vi "Example_Manifold Learning.vi"() -> ()   [LabVIEW 2020]
uses:
  <vilib>/Utility/miscctls.llb/LV3DPointTypeDef.ctl
  <vilib>/addons/Machine Learning/Utilities/ml_Neighborhood Graph_Para.ctl
  <vilib>/addons/Machine Learning/Visualization/Visualization (3D).vi
  <vilib>/addons/Machine Learning/Visualization/Visualization (2D).vi
  <vilib>/addons/Machine Learning/NILabs_MLT.lvlib
panel:
  in  "# of samples":i32=1024
  in  "Data set":enum16{"swiss roll", "hemisphere", "3 balls"}(ring)=3
  in  "Algorithm":T1(ring)
  out "2-D Projections of the data":cluster{"X":dbl[], "Y":dbl[]}[](graph)
  out "error out":errorcluster
  out "3-D Data":refnum<vi>(3d-picture)
  # "Introduction:\nA list of dimension reduction algorithms can be selected to project several 3-D data to 2-D space. Some of the data sets (e.g., swiss roll) represent 2-D manifolds embedded in 3-D space. Their underlying structure can be correctly revealed in the projection when a suitable algorithm is selected."
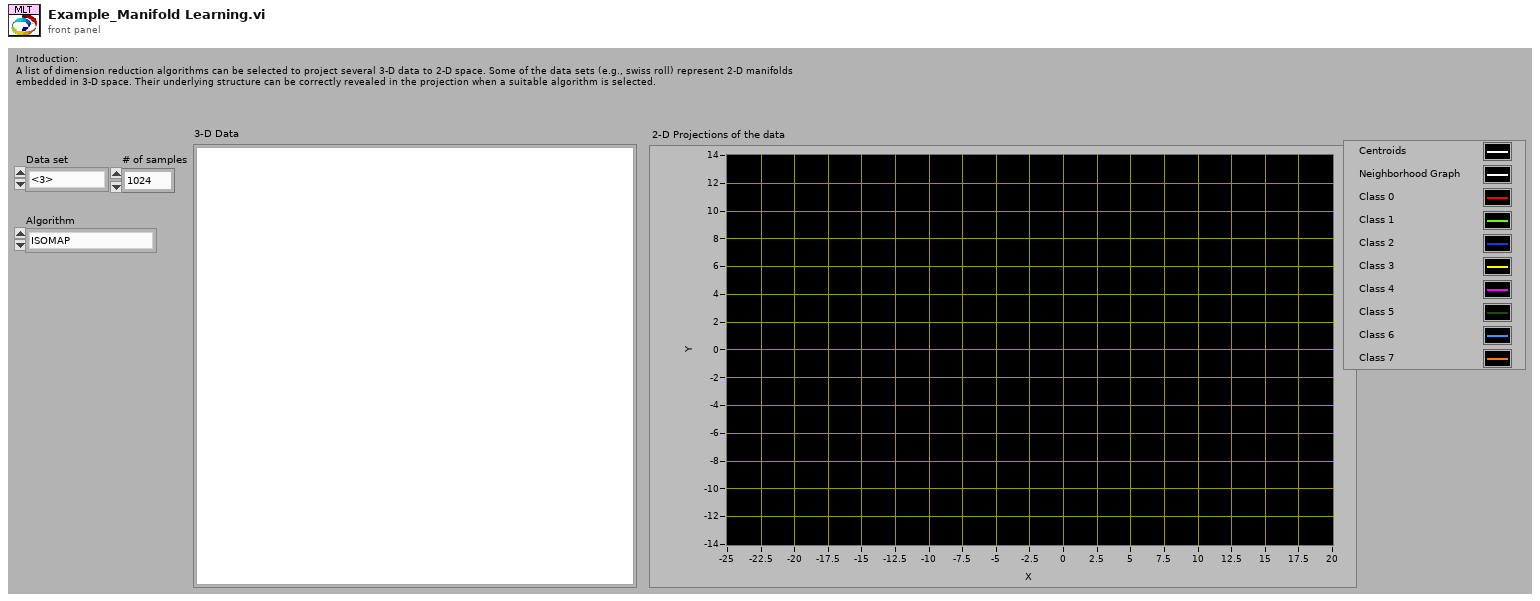
[diagram p1: front panel]
types:
  T1 = enum16{"ISOMAP", "Locally-Linear Embedding (LLE)", "PCA", "MDS", "LDA"}
  T2 = typedef "LV3DPointTypeDef.ctl" = cluster{"X":sgl, "Y":sgl, "Z":sgl}
  T3 = typedef "NILabs_MLT.lvlib/ml_Neighborhood Graph_Para.ctl" = cluster{"algorithm":enum16{"eps-Neighborhood Graph", "k-Nearest Neighbor Graph", "Mutual k-Nearest Neighbor Graph"}, "k":i32, "eps":dbl}
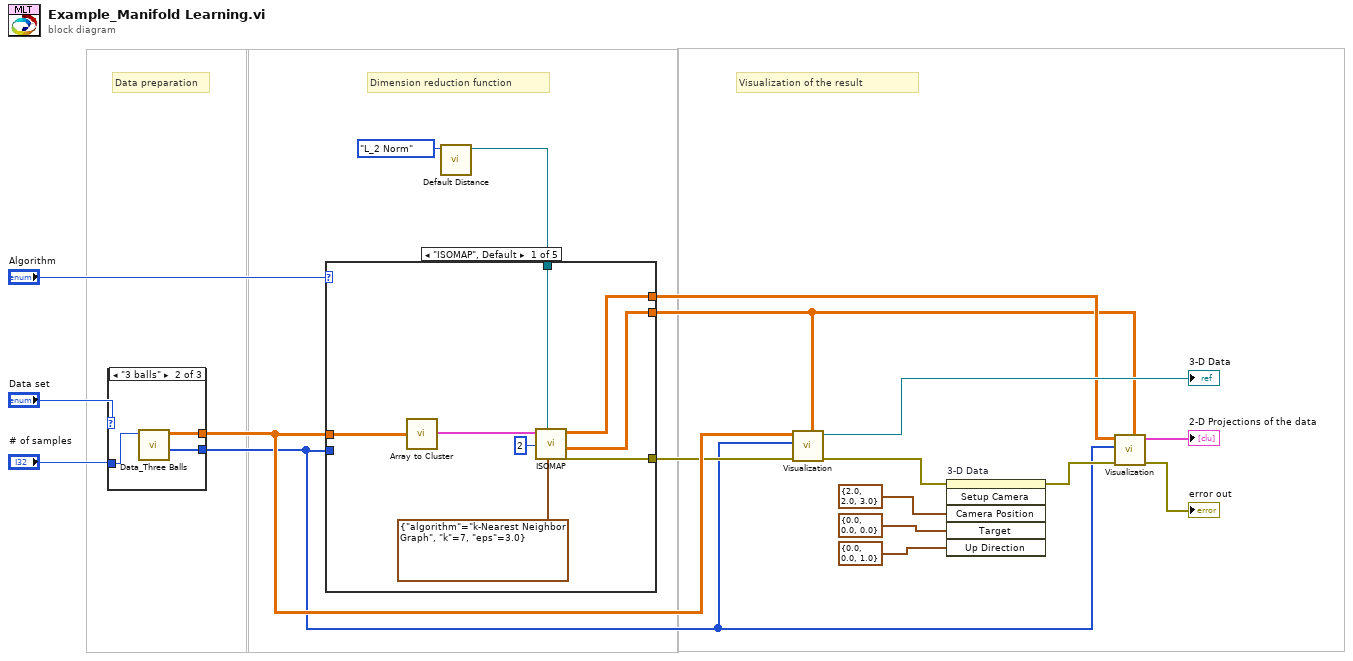
[diagram p0: block diagram]
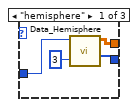
[diagram p2: hidden frame]
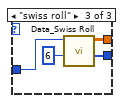
[diagram p3: hidden frame]
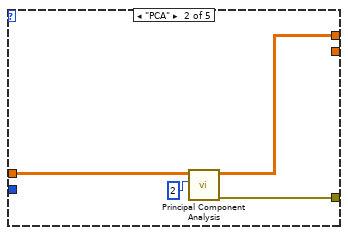
[diagram p4: hidden frame]
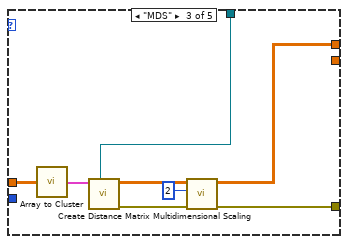
[diagram p5: hidden frame]
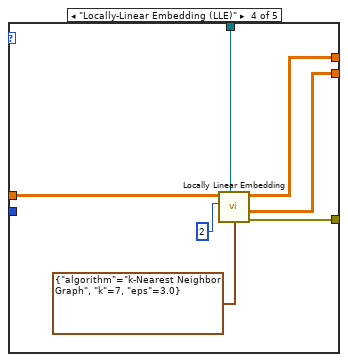
[diagram p6: hidden frame]
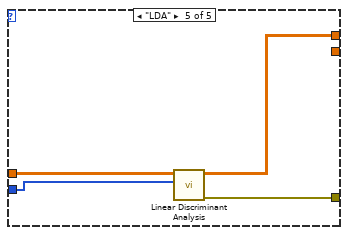
[diagram p7: hidden frame]
diagram:
  # "Visualization of the result"
  # "Dimension reduction function"
  # "Data preparation"
  n1 = case shown="\"3 balls\"" "Data set" {
    tunnel: [w22 w24 w29] -> w14
    tunnel: [w21 w23 w28] -> w1
    tunnel: "# of samples" -> [w19 w25 w26]
    frame "hemisphere" {
      n2 = call "Data_Hemisphere.vi"("# of classes"=3, "# of samples"=w19) -> ("Class labels"=w21:i32[], "Data samples"=w22:dbl[][])  [unwired: 8 in]
    }
    frame "3 balls" {
      n3 = call "Data_Three Balls.vi"("# of points"=w25) -> ("Classes"=w23:i32[], "Data"=w24:dbl[][])  [unwired: 9 in]
    }
    frame "swiss roll" {
      n4 = call "Data_Swiss Roll.vi"("# of classes"=6, "# of points"=w26) -> ("class"=w28:i32[], "Data"=w29:dbl[][])  [unwired: 8 in]
    }
  }
  n5 = call <vilib>:"Default Distance.vi"("distance norm type"=enum16{"L_1 Norm", "L_2 Norm", "L_inf Norm"}."L_2 Norm" ("norm type")) -> ("Distance VI"=w4:refnum<vi>)  [unwired: 9 in, 1 out]
  n6 = case shown="\"ISOMAP\", Default" "Algorithm" {
    tunnel: w14 -> [w37 w38 w45 w53 w60]
    tunnel: [w35 w39 w48 w56 w58] -> w13
    tunnel: [w34 w40 w47 w54 w57] -> w10
    tunnel: [w33 _ _ w55 _] -> w7
    tunnel: w4 -> [w32 _ w46 w52 _]
    tunnel: w1 -> [_ _ _ _ w59]
    frame "ISOMAP", Default {
      n7 = call <vilib>:"Array to Cluster.vi"("Data in Array"=w37) -> ("Data in Cluster"=w36:cluster{"Sample":dbl[]}[])
      n8 = call <vilib>:"ISOMAP.vi"("Neighborhood Graph Para"=T3 {"algorithm"=enum."k-Nearest Neighbor Graph", "k"=7, "eps"=3.0} ("Neighborhood Graph Parameters"), "Distance VI"=w32, "dim"=2, "Data samples"=w36) -> ("error out"=w34:errorcluster, "Neighborhood Graph"=w33:dbl[][], "Embedding"=w35:dbl[][])  [unwired: 4 in, 1 out]
    }
    frame "PCA" {
      n9 = call <vilib>:"Principal Component Analysis.vi"("dim"=2, "Data samples"=w38) -> ("error out"=w40:errorcluster, "principle components"=w39:dbl[][])  [unwired: 6 in, 2 out]
    }
    frame "MDS" {
      n10 = call <vilib>:"Array to Cluster.vi"("Data in Array"=w45) -> ("Data in Cluster"=w44:cluster{"Sample":dbl[]}[])
      n11 = call <vilib>:"Create Distance Matrix.vi"("Distance VI"=w46, "Data samples"=w44) -> ("error out"=w42:errorcluster, "Distance Matrix"=w43:dbl[][])  [unwired: 8 in]
      n12 = call <vilib>:"Multidimensional Scaling.vi"("error in (no error)"=w42, "dim"=2, "Distance"=w43) -> ("error out"=w47:errorcluster, "Embedding"=w48:dbl[][])  [unwired: 5 in, 2 out]
    }
    frame "Locally-Linear Embedding (LLE)" {
      n13 = call <vilib>:"Locally Linear Embedding.vi"("Neighborhood Graph Para"=T3 {"algorithm"=enum."k-Nearest Neighbor Graph", "k"=7, "eps"=3.0} ("Neighborhood Graph Parameters"), "Distance VI"=w52, "dim"=2, "Data samples"=w53) -> ("error out"=w54:errorcluster, "Neighborhood Graph"=w55:dbl[][], "Embedding"=w56:dbl[][])  [unwired: 4 in, 1 out]
    }
    frame "LDA" {
      n14 = call <vilib>:"Linear Discriminant Analysis.vi"("Class labels"=w59, "Examples"=w60) -> ("error out"=w57:errorcluster, "Projected Examples"=w58:dbl[][])  [unwired: 7 in, 1 out]
    }
  }
  n15 = call-poly <vilib>:"Visualization.vi"("Neighborhood Graph"=w7, "error in (no error)"=w10, "Class labels"=w1, "Data samples"=w14) -> ("error out"=w12:errorcluster, "3D Picture"=→"3-D Data":refnum<vi>)  [unwired: 6 in]
  n16 = invoke on="3-D Data" class="SceneGraphDisp (strict)" method="Setup Camera"(error in=w12, "Camera Position"=T2 {"X"=2.0, "Y"=2.0, "Z"=3.0}, "Target"=T2 {"X"=0.0, "Y"=0.0, "Z"=0.0} ("Camera Position"), "Up Direction"=T2 {"X"=0.0, "Y"=0.0, "Z"=1.0} ("Camera Position")) -> (error out=w11:errorcluster)  [unwired: 2 in, 5 out]
  n17 = call-poly <vilib>:"Visualization.vi"("Neighborhood Graph"=w7, "error in (no error)"=w11, "Class labels"=w1, "Data samples"=w13) -> ("error out"=→"error out":errorcluster, "XY Graph"=→"2-D Projections of the data":cluster{"X":dbl[], "Y":dbl[]}[])  [unwired: 6 in]
